vi "Error Logger.vi"(8 "error in (no error)":errorcluster, 11 "Current VI's Path":path) -> (0 "error out":errorcluster)   [LabVIEW 2019, in "Hawkeye.lvlib"]
uses:
  Hawkeye.lvlib
  <vilib>/Utility/sysdir.llb/System Directory Type.ctl
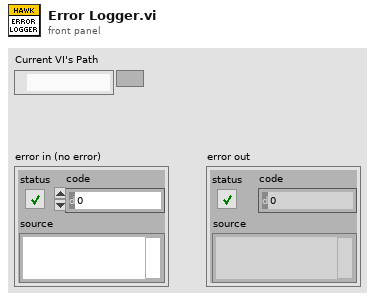
[diagram p1: front panel]
types:
  T1 = enum16{"open", "replace", "create", "open or create", "replace or create", "replace or create with confirmation"}
  T2 = typedef "System Directory Type.ctl" = i32
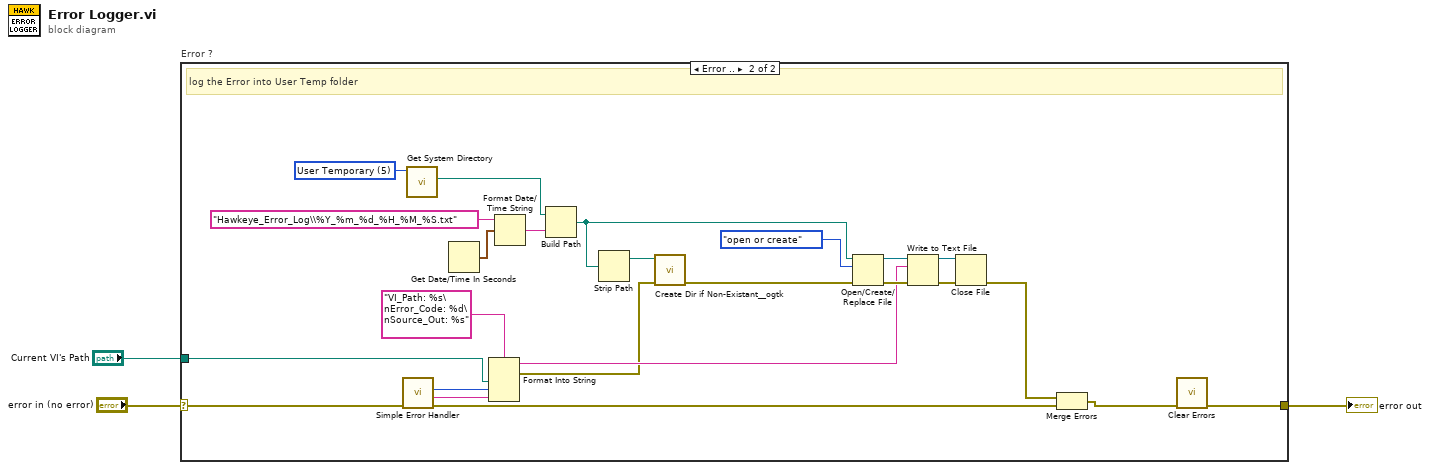
[diagram p0: block diagram]
diagram:
  n1 = case "Error ?" shown="Error .." "error in (no error)" {
    selector: "error in (no error)" -> [w4 w27]
    tunnel: [w4 w26] -> w2
    tunnel: "Current VI's Path" -> [_ w5]
    frame No Error {
      # "No error"
    }
    frame Error {
      w25 = T2 5 items=["User Home"=0, "User Desktop"=1, "User Documents"=2, "User Application Data"=3, "User Preferences"=4, "User Temporary"=5, "Public Documents"=6, "Public Application Data"=7, "Public Preferences"=8, "Public Cache"=13, "System Core Libraries"=9, "System Installed Libraries"=10, "Application Files"=11, "Boot Volume Root"=12] ("system directory type")
      # "log the Error into User Temp folder"
      n2 = call <vilib>:"Simple Error Handler.vi"("error in (no error)"=w27) -> ("code out"=w14:i32, "source out"=w13:string, "error out"=w28:errorcluster)  [unwired: 4 in, 2 out]
      n3 = call <vilib>:"Get System Directory.vi"("system directory type"=w25) -> ("system directory"=w24:path)  [unwired: 10 in]
      n4 = Get Date/Time In Seconds() -> (seconds since 1Jan1904=w22:timestamp)
      n5 = Format Into String(format string="VI_Path: %s\nError_Code: %d\nSource_Out: %s", w5, w14, w13) -> (resulting string=w12:string, error out=w8:errorcluster)  [unwired: 2 in]
      n6 = Format Date/Time String(time format string (%c)="Hawkeye_Error_Log\\%Y_%m_%d_%H_%M_%S.txt", seconds (now)=w22) -> (date/time string=w21:string)  [unwired: 1 in]
      n7 = Build Path(base path=w24, name or relative path=w21) -> (appended path=w7:path)
      n8 = Strip Path(path=w7) -> (stripped path=w6:path)  [unwired: 1 out]
      n9 = call <userlib>:"Create Dir if Non-Existant__ogtk.vi"("error in (no error)"=w8, "Directory Path"=w6) -> ("error out"=w9:errorcluster)  [unwired: 7 in, 2 out]
      n10 = Open/Create/Replace File(file path (use dialog)=w7, error in=w9, operation (0:open)=T1."open or create") -> (refnum out=w19:refnum<file>, error out=w18:errorcluster)  [unwired: 3 in, 1 out]
      n11 = Write to Text File(file (use dialog)=w19, text=w12, error in=w18) -> (refnum out=w16:refnum<file>, error out=w17:errorcluster)  [unwired: 1 in, 1 out]
      n12 = Close File(refnum=w16, error in=w17) -> (error out=w10:errorcluster)  [unwired: 1 out]
      n13 = Merge Errors(w10, w28) -> (w11:errorcluster)
      n14 = call <vilib>:"Clear Errors.vi"("error in (no error)"=w11) -> ("error out"=w26:errorcluster)  [unwired: 5 in, 1 out]
    }
  }
  "error out" <- w2
